vi "Test_sqlite3QueryVIM1DIntegerWorks_NoError.vi"(8 "error in (no error)":errorcluster, 11 "TestCase in":refnum<class "Test sqlite3.lvclass">) -> (0 "error out":errorcluster, 3 "TestCase out":refnum<class "Test sqlite3.lvclass">)   [LabVIEW 2020, in "Test sqlite3.lvclass"]
uses:
  Test sqlite3.lvclass
  externals/sqlite3/Source/sqlite3.lvclass/sqlite3.ctl
  45a547b6-e4c0-49d6-ab78-a1d3563bf804.vi
  45a547b6-e4c0-49d6-ab78-a1d3563bf804.vi/38eccb0c-c074-450d-8d15-23d2a0b1a6d9.vi
  45a547b6-e4c0-49d6-ab78-a1d3563bf804.vi/6b7cd650-cf7b-44ca-aedf-d29df7752792.vi
  <vilib>/Utility/error.llb/Error Cluster From Error Code.vi
  externals/sqlite3/Source/sqlite3.lvclass
  <vilib>/addons/_JKI Toolkits/VI Tester/TestCase.llb/TestCase.lvclass
  externals/database-interface/IDatabase/IDatabase/IDatabase.lvclass
  C:/Program Files/National Instruments/LabVIEW 2020/vi.lib/addons/_JKI Toolkits/VI Tester/TestCase.llb/TestCase.lvclass
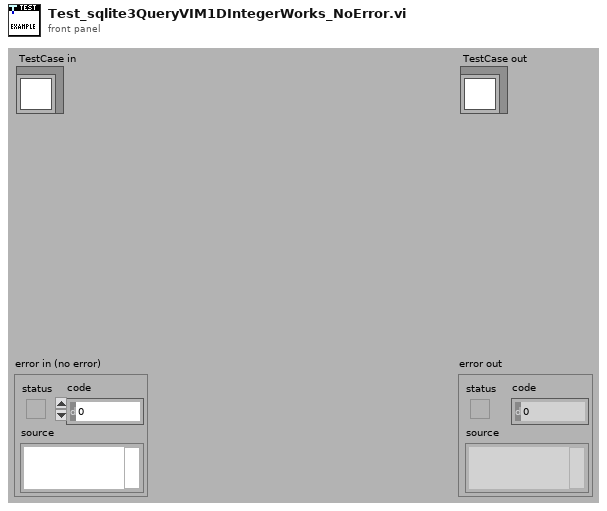
[diagram p1: front panel]
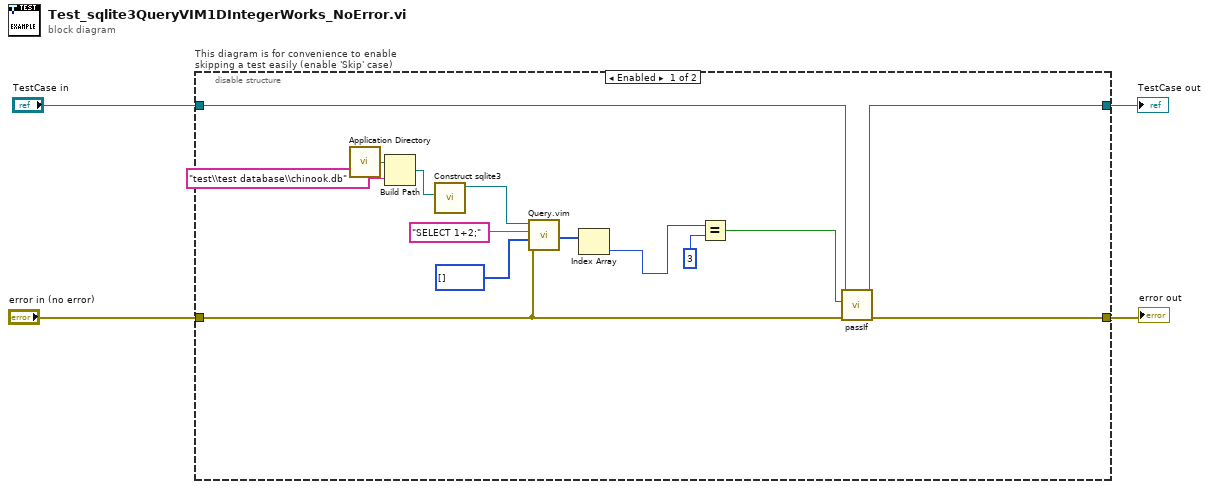
[diagram p0: block diagram]
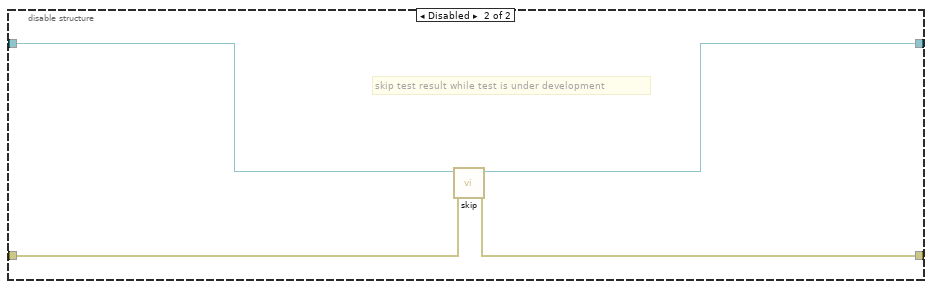
[diagram p2: hidden frame]
diagram:
  n1 = disable-structure "This diagram is for convenience to enable skipping a test easily (enable 'Skip' case)" shown="Enabled" {
    disable-tunnel: "TestCase in" -> [w16 w22]
    disable-tunnel: [w18 w20] -> w1
    disable-tunnel: [w17 w21] -> w3
    disable-tunnel: "error in (no error)" -> [w15 w19]
    frame Enabled {
      n2 = call <vilib>:"Application Directory.vi"() -> ("Application Directory"=w11:path)
      n3 = Build Path(base path=w11, name or relative path="test\\test database\\chinook.db") -> (appended path=w12:path)
      n4 = call "Construct sqlite3.vi"("DatabaseFilePath"=w12) -> ("sqlite3 out"=w7:refnum<class "sqlite3.lvclass">)  [unwired: 9 in, 1 out]
      n5 = call "Query.vim"("error in (no error)"=w15, "Type and Default"=i32[] [] ("y"), "Query string"="SELECT 1+2;", "IDatabase in"=w7) -> ("Result"=w14:i32[])  [unwired: 5 in, 2 out]
      n6 = Index Array(array=w14) -> (element=w6:i32)  [unwired: 1 in]
      n7 = Equal?(x=w6, y=3) -> (x = y?=w13:bool)
      n8 = call-dynamic "passIf.vi"("error in (no error)"=w15, "pass"=w13, "TestCase in"=w16) -> ("error out"=w17:errorcluster, "TestCase out"=w18:refnum<class "Test sqlite3.lvclass">)  [unwired: 7 in]
    }
    frame Disabled {
      # "skip test result while test is under development"
      n9 = call <vilib>:"skip.vi"("error in (no error)"=w19, "TestCase in"=w22) -> ("error out"=w21:errorcluster, "TestCase out"=w20:refnum<class "Test sqlite3.lvclass">)  [unwired: 8 in]
    }
  }
  "error out" <- w3
  "TestCase out" <- w1
